vi "复件 复件 复件 二维 扩散 最新.vi"(1 "数组 2":i16[][](array[numeric])) -> (0 "数组":i32[][](array[numeric]))   [LabVIEW 2014]
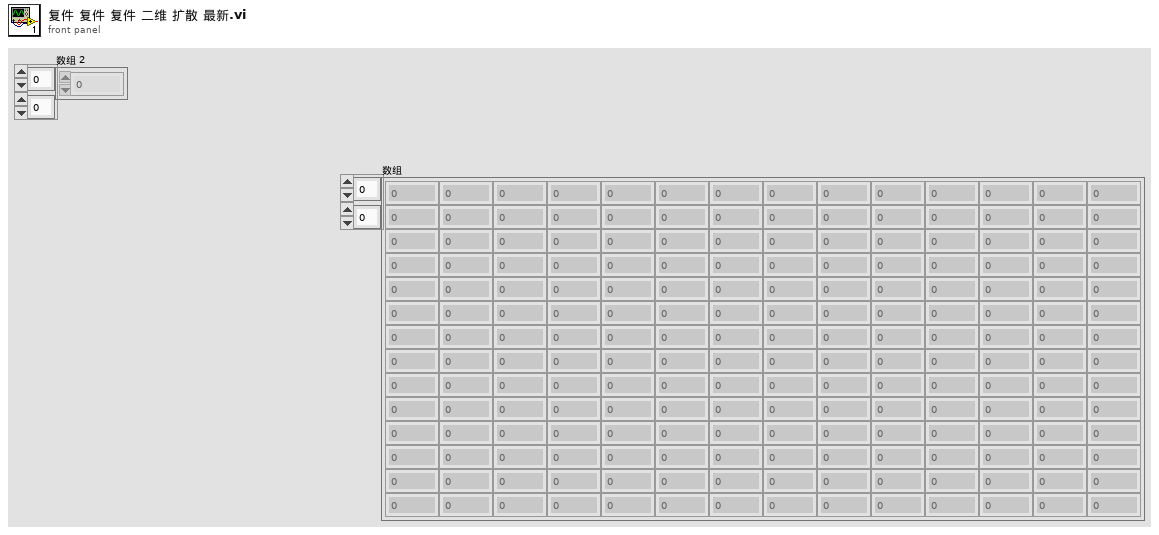
[diagram p1: front panel]
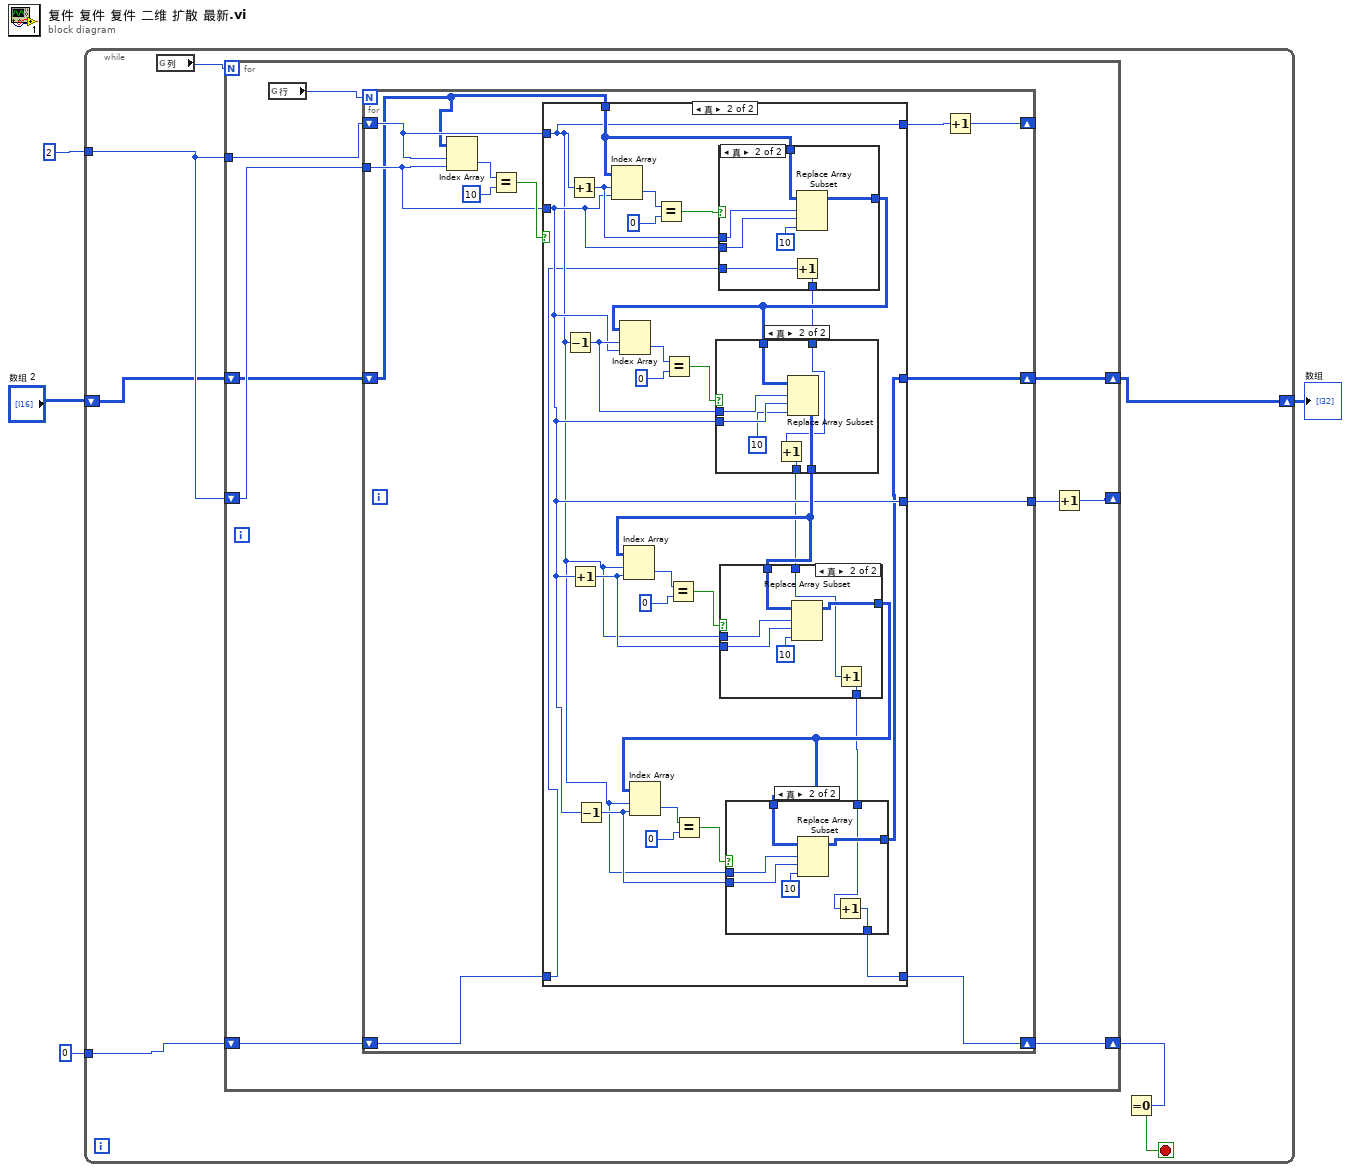
[diagram p0: block diagram]
diagram:
  n1 = while {
    tunnel: 2 -> [w9]
    shift-right: [w8] -> w3
    shift-left: "数组 2" -> [w7]
    tunnel: 0 -> [w6]
    stop <- w10 stop-if-true
    n2 = global read "全局 1.vi" "列"() -> (w5:i32)
    n3 = for {
      N: w5 -> [_]
      tunnel: w9 -> [w20]
      shift-right: [w17] -> _
      shift-left: w9 -> [w19]
      shift-right: [w16] -> w11
      shift-left: w6 -> [w15]
      shift-right: [w14] -> w8
      shift-left: w7 -> [w13]
      n4 = global read "全局 1.vi" "行"() -> (w12:i32)
      n5 = for {
        N: w12 -> [_]
        tunnel: w19 -> [w29]
        shift-right: [w28] -> w14
        shift-left: w13 -> [w23]
        shift-right: [w26] -> _
        shift-left: w20 -> [w25]
        tunnel: [w24] -> w18
        shift-right: [w22] -> w16
        shift-left: w15 -> [w21]
        n6 = Index Array(array=w23, index (row)=w25, index (col)=w29) -> (element=w32:i16)
        n7 = Equal?(x=w32, y=10) -> (x = y?=w30:bool)
        n8 = case shown="真" w30 {
          tunnel: w25 -> [w35 w43]
          tunnel: w29 -> [w34 w44]
          tunnel: w23 -> [w36 w61]
          tunnel: [w36 w42] -> w28
          tunnel: [w35 w43] -> w27
          tunnel: [w34 w44] -> w24
          tunnel: w21 -> [w33 w41]
          tunnel: [w33 w37] -> w22
          frame False {
          }
          frame True {
            n9 = Decrement(x=w43) -> (x-1=w55:i32)
            n10 = Increment(x=w43) -> (x+1=w60:i32)
            n11 = Increment(x=w44) -> (x+1=w50:i32)
            n12 = Decrement(x=w44) -> (x-1=w46:i32)
            n13 = Index Array(array=w61, index (row)=w60, index (col)=w44) -> (element=w64:i16)
            n14 = Equal?(x=w64, y=0) -> (x = y?=w62:bool)
            n15 = case shown="真" w62 {
              tunnel: w61 -> [w93 w100]
              tunnel: w60 -> [_ w99]
              tunnel: w44 -> [_ w98]
              tunnel: [w93 w96] -> w57
              tunnel: w41 -> [w92 w95]
              tunnel: [w92 w94] -> w40
              frame False {
              }
              frame True {
                n16 = Increment(x=w95) -> (x+1=w94:i32)
                n17 = Replace Array Subset(array=w100, new element=10, index (row)=w99, index (col)=w98) -> (w96:i16[][])
              }
            }
            n18 = Index Array(array=w57, index (row)=w55, index (col)=w44) -> (element=w59:i16)
            n19 = Equal?(x=w59, y=0) -> (x = y?=w56:bool)
            n20 = case shown="真" w56 {
              tunnel: w57 -> [w84 w91]
              tunnel: w55 -> [_ w90]
              tunnel: w44 -> [_ w89]
              tunnel: [w84 w87] -> w51
              tunnel: w40 -> [w83 w86]
              tunnel: [w83 w85] -> w39
              frame False {
              }
              frame True {
                n21 = Increment(x=w86) -> (x+1=w85:i32)
                n22 = Replace Array Subset(array=w91, new element=10, index (row)=w90, index (col)=w89) -> (w87:i16[][])
              }
            }
            n23 = Index Array(array=w51, index (row)=w43, index (col)=w50) -> (element=w52:i16)
            n24 = Equal?(x=w52, y=0) -> (x = y?=w53:bool)
            n25 = case shown="真" w53 {
              tunnel: w51 -> [w75 w82]
              tunnel: w43 -> [_ w81]
              tunnel: w50 -> [_ w80]
              tunnel: [w75 w78] -> w45
              tunnel: w39 -> [w74 w77]
              tunnel: [w74 w76] -> w38
              frame False {
              }
              frame True {
                n26 = Replace Array Subset(array=w82, new element=10, index (row)=w81, index (col)=w80) -> (w78:i16[][])
                n27 = Increment(x=w77) -> (x+1=w76:i32)
              }
            }
            n28 = Index Array(array=w45, index (row)=w43, index (col)=w46) -> (element=w47:i16)
            n29 = Equal?(x=w47, y=0) -> (x = y?=w48:bool)
            n30 = case shown="真" w48 {
              tunnel: w45 -> [w66 w73]
              tunnel: w43 -> [_ w72]
              tunnel: w46 -> [_ w71]
              tunnel: [w66 w69] -> w42
              tunnel: w38 -> [w65 w68]
              tunnel: [w65 w67] -> w37
              frame False {
              }
              frame True {
                n31 = Replace Array Subset(array=w73, new element=10, index (row)=w72, index (col)=w71) -> (w69:i16[][])
                n32 = Increment(x=w68) -> (x+1=w67:i32)
              }
            }
          }
        }
        n33 = Increment(x=w27) -> (x+1=w26:i32)
      }
      n34 = Increment(x=w18) -> (x+1=w17:i32)
    }
    n35 = Equal To 0?(x=w11) -> (x = 0?=w10:bool)
  }
  "数组" <- w3
